vi "Sever SSL.vi"() -> ()   [LabVIEW 2014]
uses:
  <userlib>/SSL Library/Controls/SSL_Data.ctl
  <userlib>/SSL Library/Controls/Ref.ctl
  <userlib>/SSL Library/SSL Lib.lvlib
panel:
  out "Listener Ref":refnum<k24>
  out "Client Connected ?":bool
  in  "Ssl Protocols Type":i32(ring)=240 items=["None"=0, "Ssl2"=12, "Ssl3"=48, "Tls"=192, "Default"=240]
  in  "Client Certificate Required":bool
  in  "Input Message":string="keep alive,30000;" caption="Type Message to send"
  out "Message Read":string
  in  "Port Number":i32=4001
  out "Status":string
  in  "Stop Button":bool
  in  "Restart":bool
  in  "Read":bool
  in  "Write":bool
  out "Error Out":errorcluster
  in  "Password":string="password"
  in  "Certificate Path":string="E:\\Work_D\\Projects\\Otis\\Backup\\SSL\\Certificates\\MyServer.pfx"
  in  "Error In":errorcluster
  # "TCP Server over SSL"
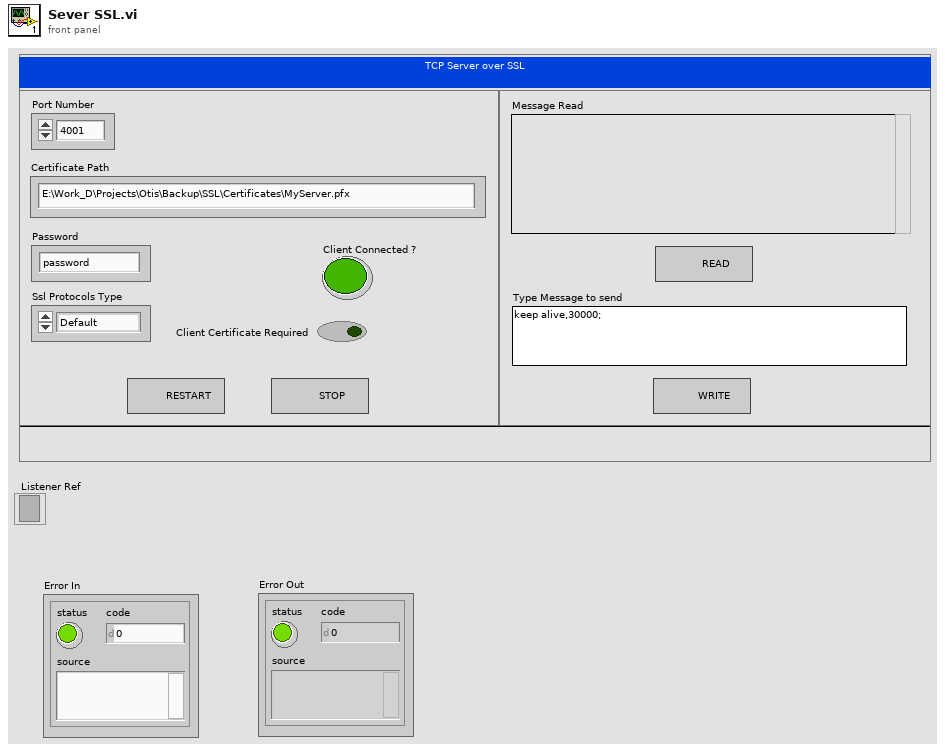
[diagram p1: front panel]
types:
  T1 = typedef "SSL_Data.ctl" = cluster{"Listener Ref":refnum<k24>, "Certificate":refnum<k24>, "AcceptTcpClient":refnum<k24>, "SSL Stream":refnum<k24>, "Message Read":string}
  T2 = enum16{"Poll", "Open Listener", "Generate Certificate", "Wait for Client", "Open SSL Steram", "Read from SSL Stream", "Write Data to SSL Steram", "Close Connection"}
  T3 = typedef "Ref.ctl" = enum16{"Update Ref", "Read Ref", "Close Ref"}
  T4 = cluster{"Certificate Ref":refnum<k24>, "Client Certificate Required":bool, "Ssl Protocols Type":i32, "Check Certificate Revocation":bool}
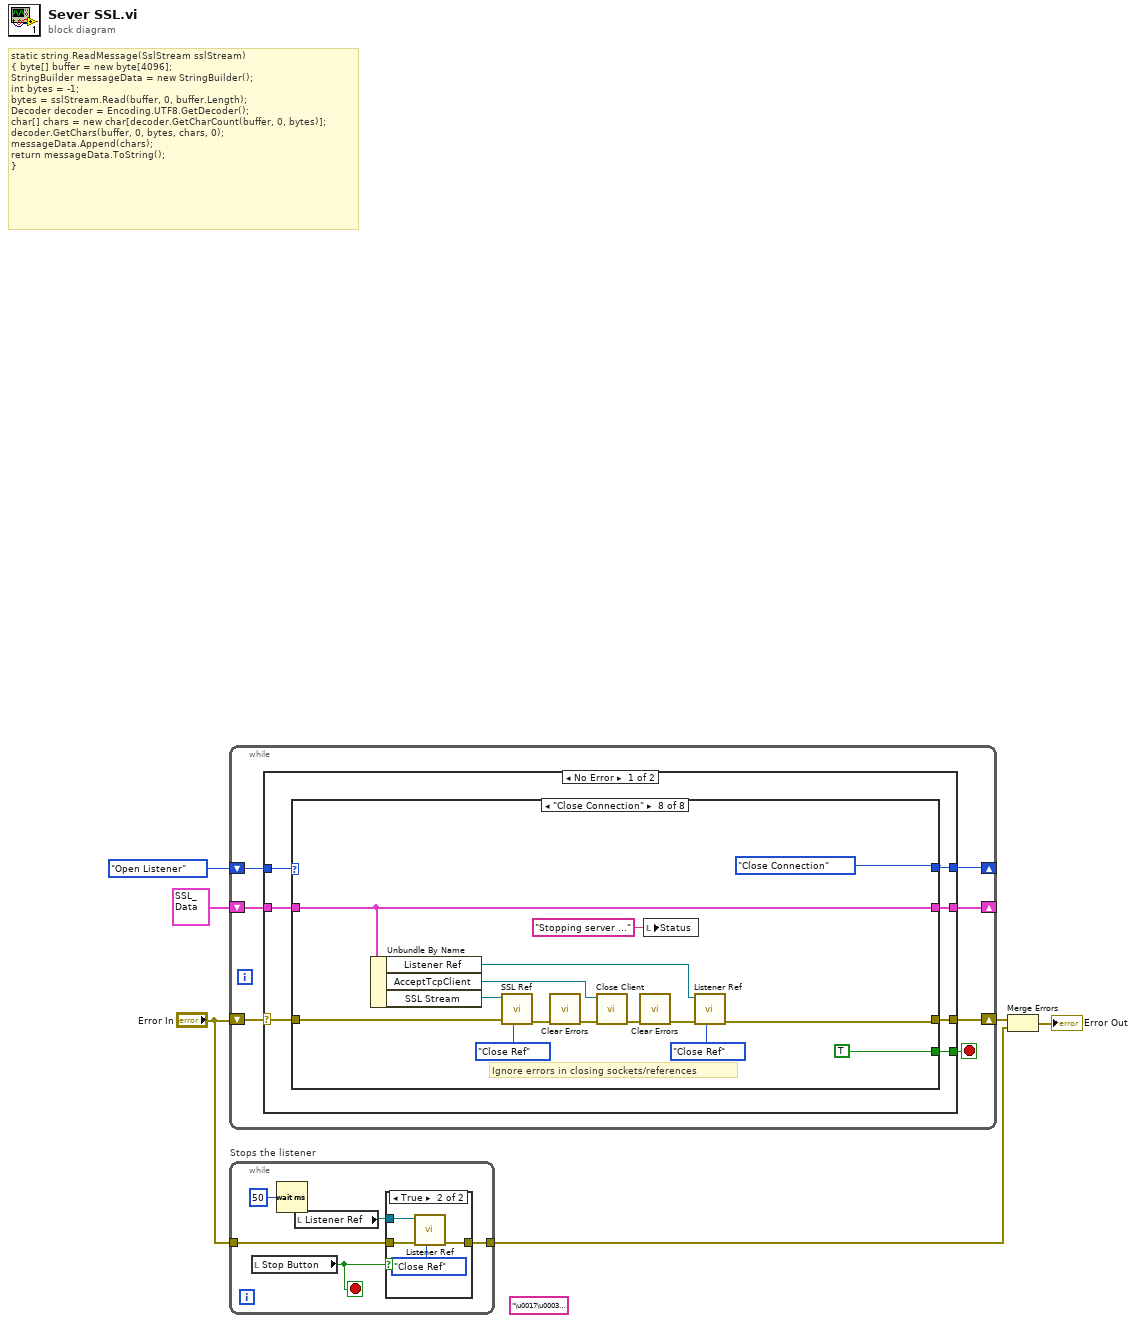
[diagram p0: block diagram]
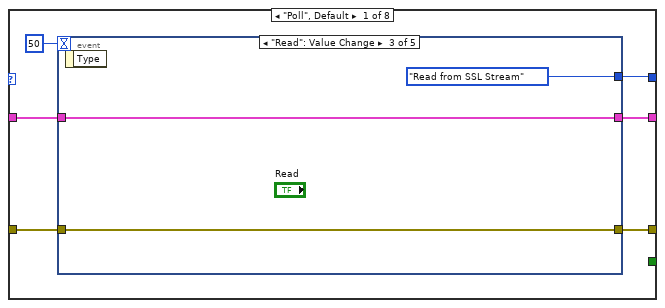
[diagram p3: hidden frame]
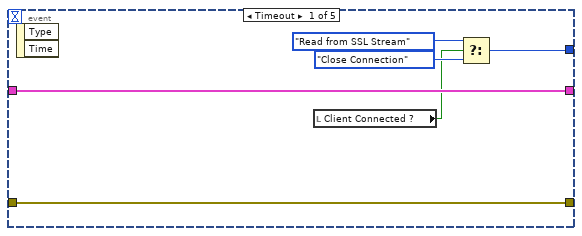
[diagram p4: hidden frame]
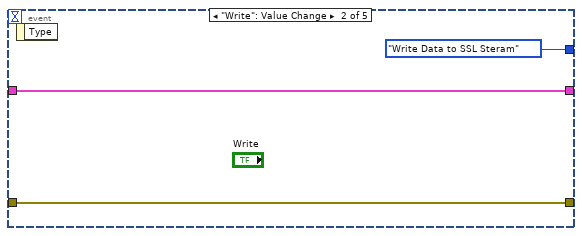
[diagram p5: hidden frame]
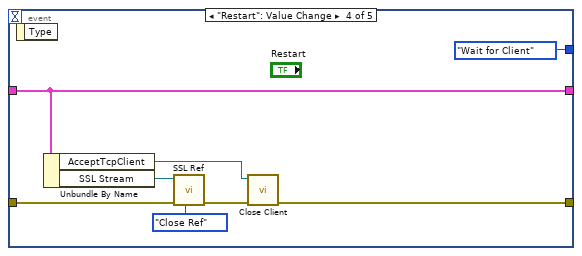
[diagram p6: hidden frame]
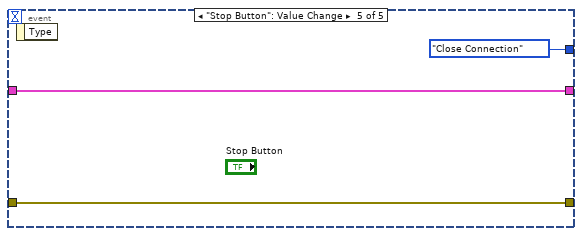
[diagram p7: hidden frame]
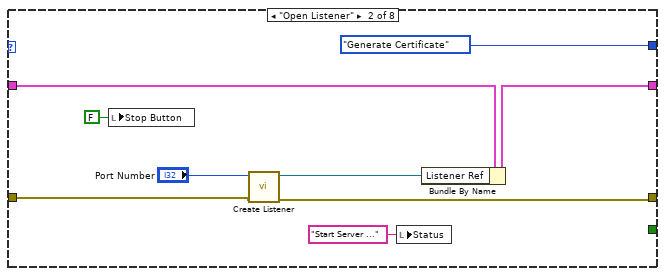
[diagram p8: hidden frame]
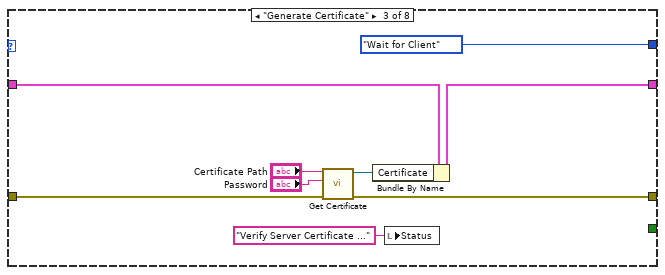
[diagram p9: hidden frame]
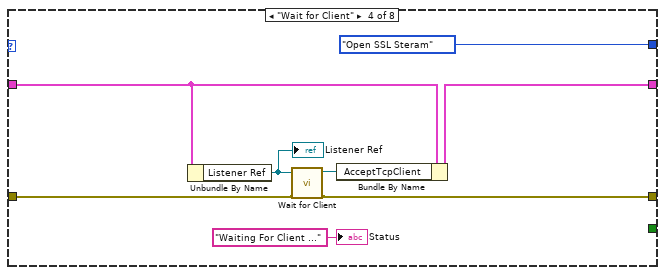
[diagram p10: hidden frame]
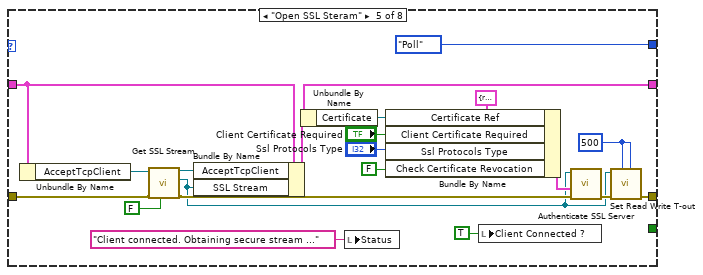
[diagram p11: hidden frame]
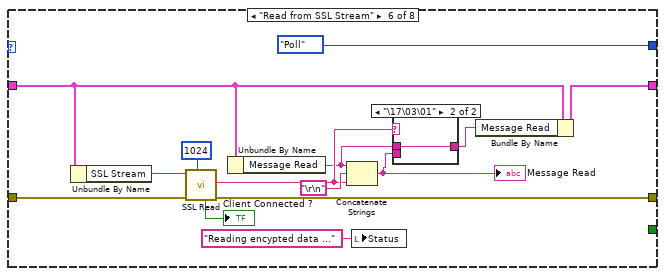
[diagram p12: hidden frame]
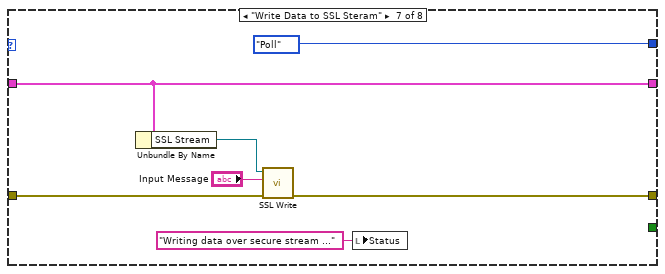
[diagram p14: hidden frame]
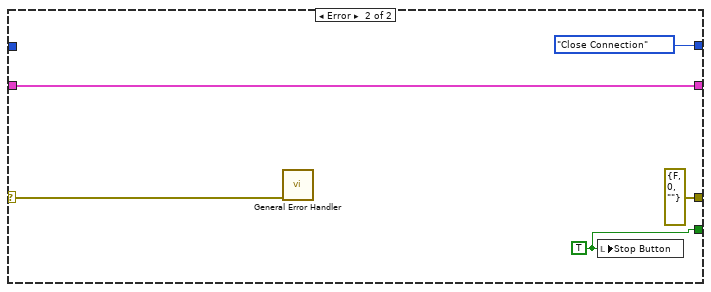
[diagram p15: hidden frame]
diagram:
  (unwired) "\u0017\u0003\u0001"
  # "static string ReadMessage(SslStream sslStream) \n{ byte[] buffer = new byte[4096];\nStringBuilder messageData = new StringBuilder(); \nint bytes = -1;\nbytes = sslStream.Read(buffer, 0, buffer.Length);\nDecoder decoder = Encoding.UTF8.GetDecoder(); \nchar[] chars = new char[decoder.GetCharCount(buffer, 0, bytes)]; \ndecoder.GetChars(buffer, 0, bytes, chars, 0); \nmessageData.Append(chars);\nreturn messageData.ToString();\n}"
  n1 = while {
    shift-right: [w11] -> _
    shift-left: T1 {"Listener Ref"=refnum, "Certificate"=refnum, "AcceptTcpClient"=refnum, "SSL Stream"=refnum, "Message Read"=""} -> [w12]
    shift-right: [w13] -> w3
    shift-left: "Error In" -> [w10]
    shift-right: [w8] -> _
    shift-left: T2."Open Listener" -> [w9]
    stop <- w7 stop-if-true
    n2 = case shown="No Error" w10 {
      selector: w10 -> [w17 w136]
      tunnel: [w20 errorcluster {"status"=FALSE, "code"=0, "source"=""} ("Error Out")] -> w13
      tunnel: w12 -> [w19 w138]
      tunnel: [w18 w138] -> w11
      tunnel: w9 -> [w16 _]
      tunnel: [w15 T2."Close Connection"] -> w8
      tunnel: [w14 w134] -> w7
      frame No Error {
        n3 = case shown="\"Close Connection\"" w16 {
          tunnel: w17 -> [w24 w57 w64 w72 w94 w108 w117 w131]
          tunnel: [w23 w56 w63 w71 w79 w107 w116 w127] -> w20
          tunnel: w19 -> [w26 w51 w67 w69 w91 w102 w114 w122]
          tunnel: [w25 w50 w66 w75 w87 w101 w114 w122] -> w18
          tunnel: [w22 T2."Generate Certificate" T2."Wait for Client" T2."Open SSL Steram" T2."Poll" T2."Poll" T2."Poll" T2."Close Connection"] -> w15
          tunnel: [_ _ _ _ _ _ _ TRUE] -> w14
          frame "Poll", Default {
            n4 = event shown="[2] \"Read\": Value Change" {
              selector: _ -> [_ _ _ _ _]
              dyn-events: _ -> [_ _ _ _ _]
              timeout: 50 -> [_ _ _ _ _]
              tunnel: w26 -> [w29 w35 w38 w41 w48]
              tunnel: [w29 w35 w38 w41 w48] -> w25
              tunnel: w24 -> [w28 w34 w37 w45 w49]
              tunnel: [w28 w34 w37 w43 w49] -> w23
              tunnel: [w32 T2."Write Data to SSL Steram" T2."Read from SSL Stream" T2."Wait for Client" T2."Close Connection"] -> w22
              event Timeout {
                n5 = event-data() -> ()  [unwired: 1 in, 2 out]
                n6 = local read "Client Connected ?"() -> (w27:bool)
                n7 = Select(t=T2."Read from SSL Stream", s=w27, f=T2."Close Connection") -> (s? t:f=w32:T2)
              }
              event "Write": Value Change {
                n8 = event-data() -> ()  [unwired: 1 in, 1 out]
              }
              event "Read": Value Change {
                n9 = event-data() -> ()  [unwired: 1 in, 1 out]
              }
              event "Restart": Value Change {
                n10 = event-data() -> ()  [unwired: 1 in, 1 out]
                n11 = Unbundle By Name(w41) -> ("AcceptTcpClient"=w39:refnum<k24>, "SSL Stream"=w40:refnum<k24>)
                n12 = call <userlib>:"SSL Ref.vi"("Action"=Ref."Close Ref", "Error In"=w45, "SSL Stream"=w40) -> ("Error Out"=w44:errorcluster)  [unwired: 7 in, 1 out]
                n13 = call <userlib>:"Close Client.vi"("Error In"=w44, "Client Ref"=w39) -> ("Error Out"=w43:errorcluster)  [unwired: 9 in]
              }
              event "Stop Button": Value Change {
                n14 = event-data() -> ()  [unwired: 1 in, 1 out]
              }
            }
          }
          frame "Open Listener" {
            n15 = local write "Stop Button"(FALSE ("Stop Button")) -> ()
            n16 = call <userlib>:"Create Listener.vi"("Error In"=w57, "Port Number"="Port Number") -> ("Error Out"=w56:errorcluster, "Listener"=w52:refnum<k24>)  [unwired: 8 in]
            n17 = local write "Status"("Start Server ..." ("Status")) -> ()
            n18 = Bundle By Name(cluster=w51, "Listener Ref"=w52) -> (w50:T1)
          }
          frame "Generate Certificate" {
            n19 = call <userlib>:"Get Certificate.vi"("Error In"=w64, "Password"="Password", "Certificate Path"="Certificate Path") -> ("Error Out"=w63:errorcluster, "Certificate"=w62:refnum<k24>)  [unwired: 6 in, 1 out]
            n20 = Bundle By Name(cluster=w67, "Certificate"=w62) -> (w66:T1)
            n21 = local write "Status"("Verify Server Certificate ..." ("Status")) -> ()
          }
          frame "Wait for Client" {
            n22 = Unbundle By Name(w69) -> ("Listener Ref"=w68:refnum<k24>)
            "Listener Ref" <- w68
            n23 = call <userlib>:"Wait for Client.vi"("Error In"=w72, "Listener Ref"=w68) -> ("Error Out"=w71:errorcluster, "Client Ref"=w70:refnum<k24>)  [unwired: 8 in]
            n24 = Bundle By Name(cluster=w69, "AcceptTcpClient"=w70) -> (w75:T1)
            "Status" <- "Waiting For Client ..." ("Status")
          }
          frame "Open SSL Steram" {
            w77 = 500 ("Read Timeout(in ms)")
            n25 = Unbundle By Name(w91) -> ("AcceptTcpClient"=w92:refnum<k24>)
            n26 = call <userlib>:"Get SSL Stream.vi"("Leave Inner Stream Open"=FALSE, "Error In"=w94, "Client Ref"=w92) -> ("Error Out"=w89:errorcluster, "SSL Ref"=w78:refnum<k24>, "Client Ref"=w90:refnum<k24>)  [unwired: 6 in]
            n27 = Bundle By Name(cluster=w91, "AcceptTcpClient"=w90, "SSL Stream"=w78) -> (w87:T1)
            n28 = Unbundle By Name(w87) -> ("Certificate"=w86:refnum<k24>)
            n29 = local write "Status"("Client connected. Obtaining secure stream ..." ("Status")) -> ()
            n30 = Bundle By Name(cluster=T4 {"Certificate Ref"=refnum, "Client Certificate Required"=FALSE, "Ssl Protocols Type"=0, "Check Certificate Revocation"=FALSE} ("Input Data"), "Certificate Ref"=w86, "Client Certificate Required"="Client Certificate Required", "Ssl Protocols Type"="Ssl Protocols Type", "Check Certificate Revocation"=FALSE) -> (w85:T4)
            n31 = local write "Client Connected ?"(TRUE ("Client Connected ?")) -> ()
            n32 = call <userlib>:"Authenticate SSL Server.vi"("Error In"=w89, "Input Data"=w85, "SSL Stream"=w78) -> ("Error Out"=w80:errorcluster)  [unwired: 8 in]
            n33 = call <userlib>:"Set Read Write T-out.vi"("Write Timeout(in ms)"=w77, "Read Timeout(in ms)"=w77, "Error In"=w80, "SSL Stream"=w78) -> ("Error Out"=w79:errorcluster)  [unwired: 7 in]
          }
          frame "Read from SSL Stream" {
            n34 = Unbundle By Name(w102) -> ("SSL Stream"=w103:refnum<k24>)
            n35 = call <userlib>:"SSL Read.vi"("Buffer Size"=1024, "Error In"=w108, "SSL Stream"=w103) -> ("Error Out"=w107:errorcluster, "Message Read"=w100:string, "Client Connected ?"=→"Client Connected ?":bool)  [unwired: 6 in]
            n36 = Unbundle By Name(w102) -> ("Message Read"=w99:string)
            n37 = Concatenate Strings(w99, "\r\n", w100) -> (w97:string)
            "Message Read" <- w97
            n38 = local write "Status"("Reading encypted data ..." ("Status")) -> ()
            n39 = case shown="\"\\17\\03\\01\"" w100 {
              tunnel: w99 -> [_ w111]
              tunnel: [w110 w111] -> w98
              tunnel: w97 -> [w110 _]
              frame "False", Default {
              }
              frame "\u0017\u0003\u0001" {
              }
            }
            n40 = Bundle By Name(cluster=w102, "Message Read"=w98) -> (w101:T1)
          }
          frame "Write Data to SSL Steram" {
            n41 = Unbundle By Name(w114) -> ("SSL Stream"=w112:refnum<k24>)
            n42 = call <userlib>:"SSL Write.vi"("Error In"=w117, "Input Message"="Input Message", "SSL Stream"=w112) -> ("Error Out"=w116:errorcluster)  [unwired: 8 in]
            n43 = local write "Status"("Writing data over secure stream ..." ("Status")) -> ()
          }
          frame "Close Connection" {
            # "Ignore errors in closing sockets/references"
            n44 = Unbundle By Name(w122) -> ("Listener Ref"=w119:refnum<k24>, "AcceptTcpClient"=w120:refnum<k24>, "SSL Stream"=w121:refnum<k24>)
            n45 = call <userlib>:"SSL Ref.vi"("Action"=Ref."Close Ref", "Error In"=w131, "SSL Stream"=w121) -> ("Error Out"=w130:errorcluster)  [unwired: 7 in, 1 out]
            n46 = call <vilib>:"Clear Errors.vi"("error in (no error)"=w130) -> ("error out"=w124:errorcluster)  [unwired: 5 in, 1 out]
            n47 = call <userlib>:"Close Client.vi"("Error In"=w124, "Client Ref"=w120) -> ("Error Out"=w128:errorcluster)  [unwired: 9 in]
            n48 = call <vilib>:"Clear Errors.vi"("error in (no error)"=w128) -> ("error out"=w123:errorcluster)  [unwired: 5 in, 1 out]
            n49 = local write "Status"("Stopping server ..." ("Status")) -> ()
            n50 = call <userlib>:"Listener Ref.vi"("Action"=Ref."Close Ref", "Error In"=w123, "Listener Ref"=w119) -> ("Error Out"=w127:errorcluster)  [unwired: 7 in, 1 out]
          }
        }
      }
      frame Error {
        w134 = TRUE
        n51 = call <vilib>:"General Error Handler.vi"("error in (no error)"=w136) -> ()  [unwired: 10 in, 5 out]
        n52 = local write "Stop Button"(w134) -> ()
      }
    }
  }
  n53 = while "Stops the listener" {
    tunnel: "Error In" -> [w142]
    tunnel: [w140] -> w2
    stop <- w143 stop-if-true
    n54 = local read "Stop Button"() -> (w143:bool)
    n55 = Wait (ms)(milliseconds to wait=u32 50) -> ()  [unwired: 1 out]
    n56 = local read "Listener Ref"() -> (w139:refnum<k24>)
    n57 = case shown="True" w143 {
      tunnel: w142 -> [w144 w147]
      tunnel: [w144 w146] -> w140
      tunnel: w139 -> [_ w145]
      frame False {
      }
      frame True {
        n58 = call <userlib>:"Listener Ref.vi"("Action"=Ref."Close Ref", "Error In"=w147, "Listener Ref"=w145) -> ("Error Out"=w146:errorcluster)  [unwired: 7 in, 1 out]
      }
    }
  }
  n59 = Merge Errors(w3, w2) -> (→"Error Out":errorcluster)
